vi "Obtain_value_selected.vi"(10 "index (row)":i32, 11 "MulticolumnListbox in":refnum<vi>) -> (3 "element":string)   [LabVIEW 2019, in "Soda_Actor.lvlib" / "Soda_Actor.lvclass"]
uses:
  Soda_Actor.lvclass
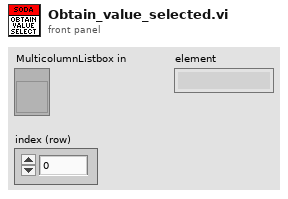
[diagram p1: front panel]
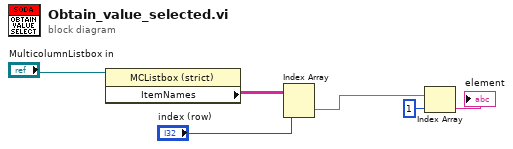
[diagram p0: block diagram]
diagram:
  n1 = property class="MCListbox (strict)"(reference="MulticolumnListbox in") -> ("ItemNames"=w2:string[][])  [unwired: 1 in, 2 out]
  n2 = Index Array(array=w2, index (row)="index (row)") -> (element=w5:string[])  [unwired: 1 in]
  n3 = Index Array(array=w5, index=1) -> (element=→"element":string)
